vi "Module Type.vi"(11 "DAQmxAO in":refnum<class "DAQmxAO.lvclass">) -> (2 "Module Type":string)   [LabVIEW 2020, in "VolatusDAQ.lvlib" / "DAQmxAO.lvclass"]
uses:
  DAQmxAO.lvclass
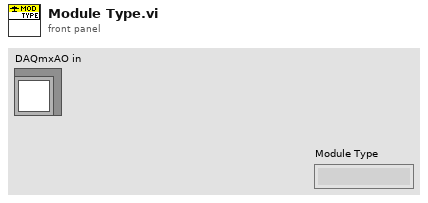
[diagram p1: front panel]
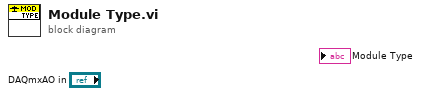
[diagram p0: block diagram]
diagram:
